vi "tlc_Stop.vi"(8 "error in":errorcluster, 11 "tlc_Consumer Queue Reference.ctl":T1) -> (0 "error out":errorcluster)   [LabVIEW 2010]
uses:
  Controls/tlc_Consumer Queue Reference.ctl
  Controls/tlc_Consumer Control.ctl
  Application Command/Application Command.lvclass
  Play/Play.lvclass
panel:
  # "Output"
  # "Input"
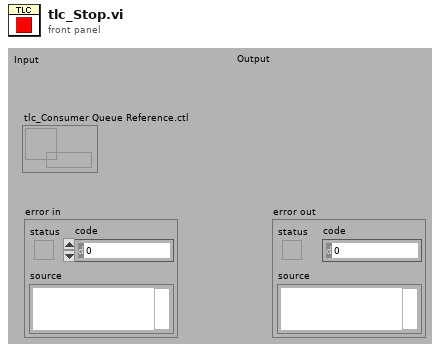
[diagram p1: front panel]
types:
  T1 = typedef "tlc_Consumer Queue Reference.ctl" = refnum<queue>
  T2 = typedef "tlc_Consumer Control.ctl" = refnum<class "Application Command.lvclass">
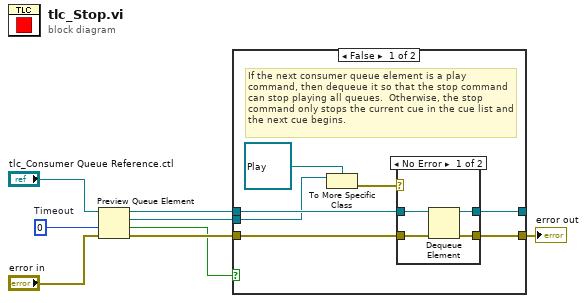
[diagram p0: block diagram]
diagram:
  w4 = 0  # Timeout
  n1 = Preview Queue Element(queue="tlc_Consumer Queue Reference.ctl", timeout in ms (-1)=w4, error in (no error)="error in") -> (queue out=w7:T1, element=w6:T2, timed out?=w5:bool, error out=w8:errorcluster)
  n2 = case shown="False" w5 {
    tunnel: w6 -> [w10 _]
    tunnel: w7 -> [w15 w23]
    tunnel: w8 -> [w14 w22]
    tunnel: [w13 w22] -> w1
    tunnel: [w12 w23] -> _
    frame False {
      # "If the next consumer queue element is a play command, then dequeue it so that the stop command can stop playing all queues.  Otherwise, the stop command only stops the current cue in the cue list and the next cue begins."
      n3 = To More Specific Class(target class=refnum<class "Play.lvclass"> refnum ("Play.lvclass"), reference=w10) -> (error out=w9:errorcluster)  [unwired: 1 in, 1 out]
      n4 = case shown="No Error" w9 {
        tunnel: w15 -> [w19 w21]
        tunnel: w14 -> [w18 w20]
        tunnel: [w17 w20] -> w13
        tunnel: [w16 w21] -> w12
        frame No Error {
          n5 = Dequeue Element(queue=w19, error in (no error)=w18) -> (queue out=w16:T1, error out=w17:errorcluster)  [unwired: 1 in, 2 out]
        }
        frame Error {
        }
      }
    }
    frame True {
    }
  }
  "error out" <- w1
